vi "AI@InstanceEditor__Parameter.vi"(1 "ParamterIn":string) -> (0 "ParamterOut":string)   [LabVIEW 2020]
uses:
  MainFrame/Global.vi
  <vilib>/vision/NI_Vision_Development_Module.lvlib
panel:
  in  "Rotate":string(combo)
  out "Image":T1(plugin-control)
  in  "Preview":bool
  in  "SubDir":string(combo)
  in  "Capture":string(combo)
  in  "Confirm":bool
  # "AI@InstanceEditor $Capture(\\$Directory)(,Rotate=1)"
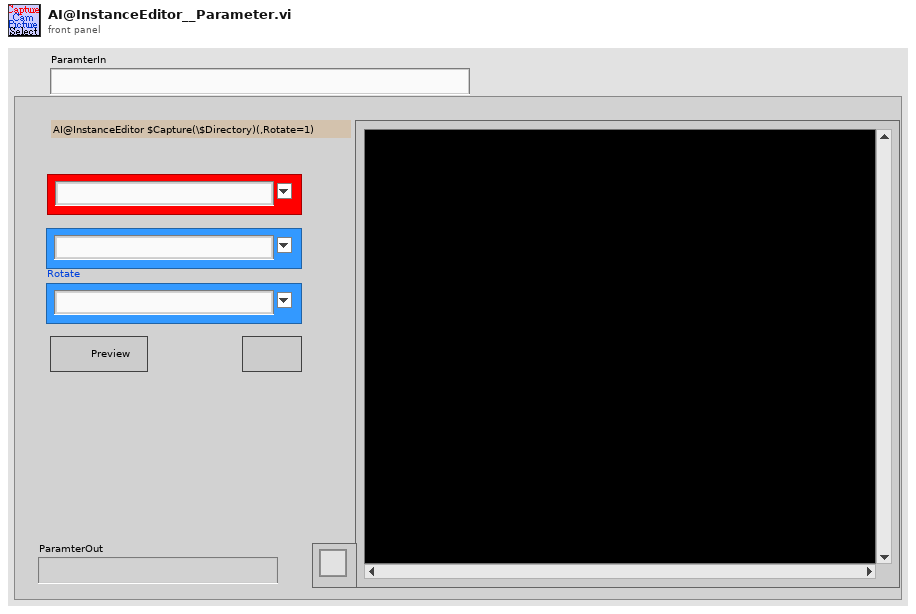
[diagram p1: front panel]
types:
  T1 = typedef "IMAQ Image.ctl" = refnum<image>
  T2 = cluster{"Browser Size":cluster{"X":i32, "Y":i32}, "Images per Line":i32, "Background Color":u32, "Frame Size":i32, "Frame Style":u16}
  T3 = typedef "Image Type" = u32
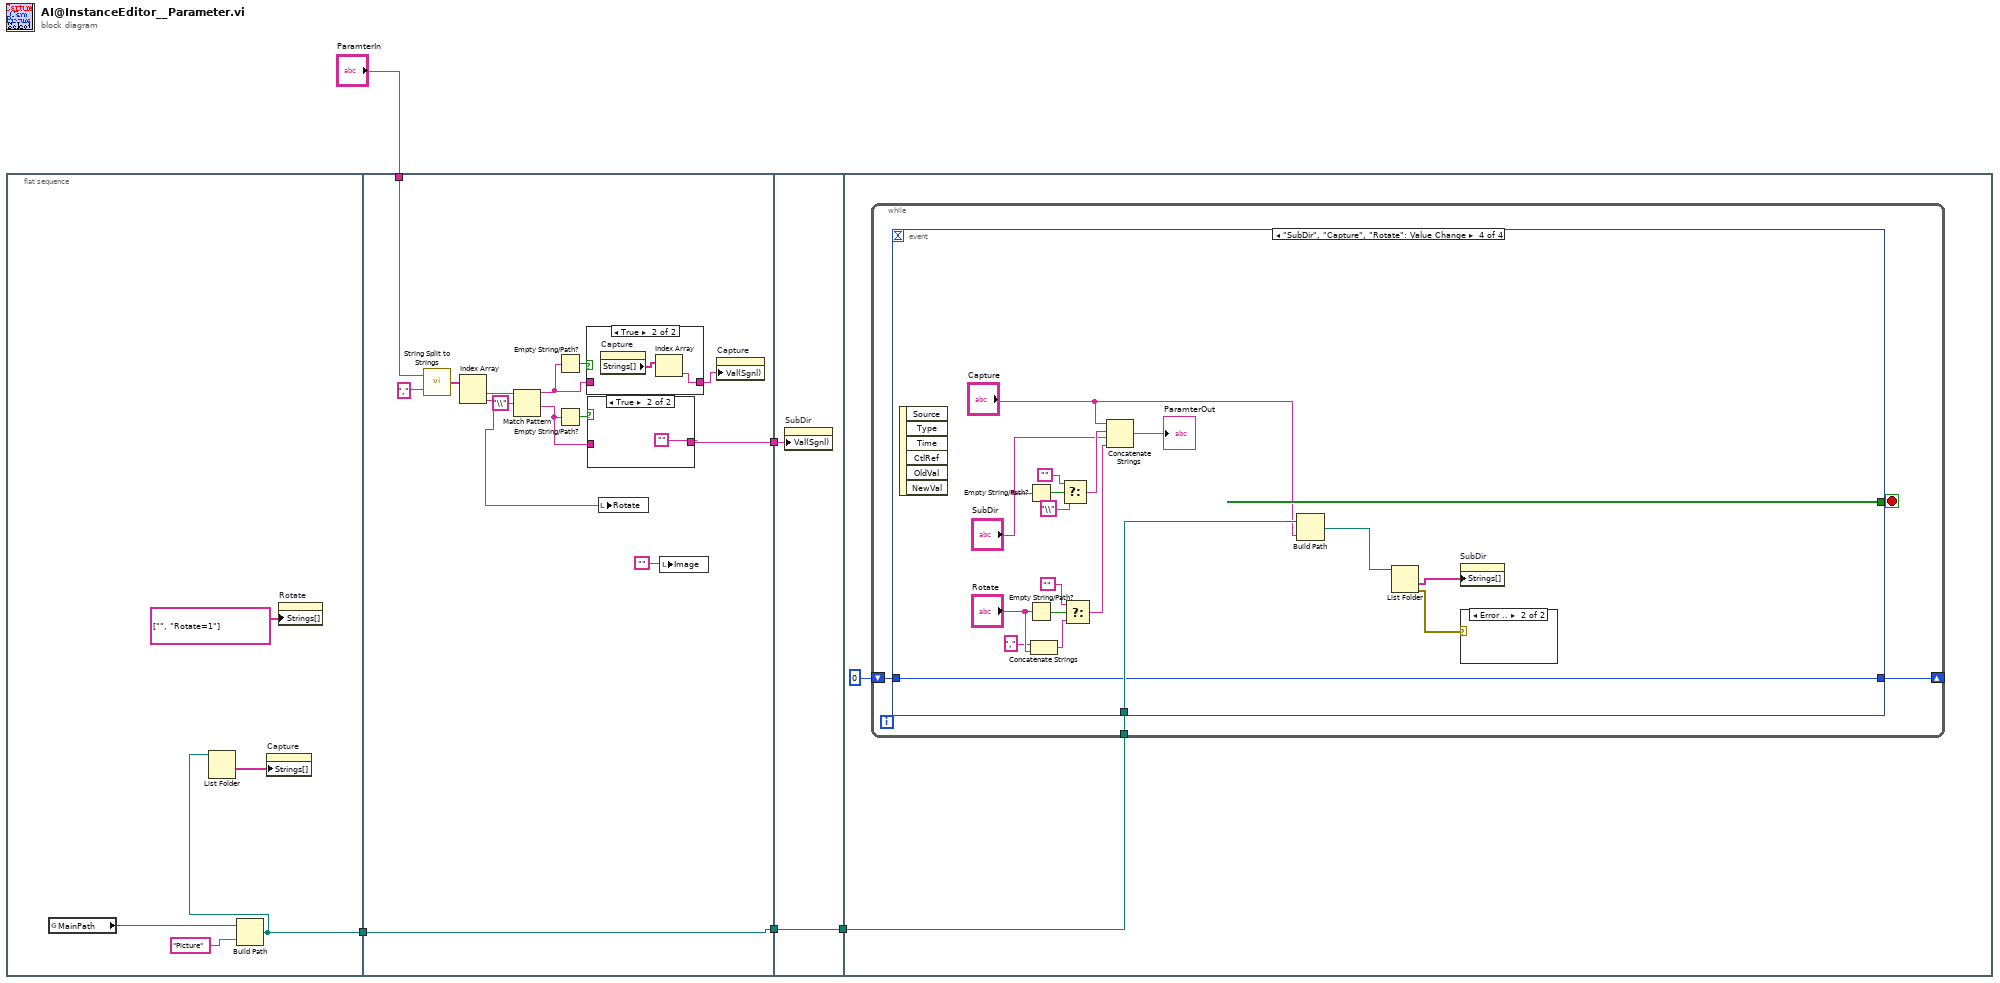
[diagram p0: block diagram]
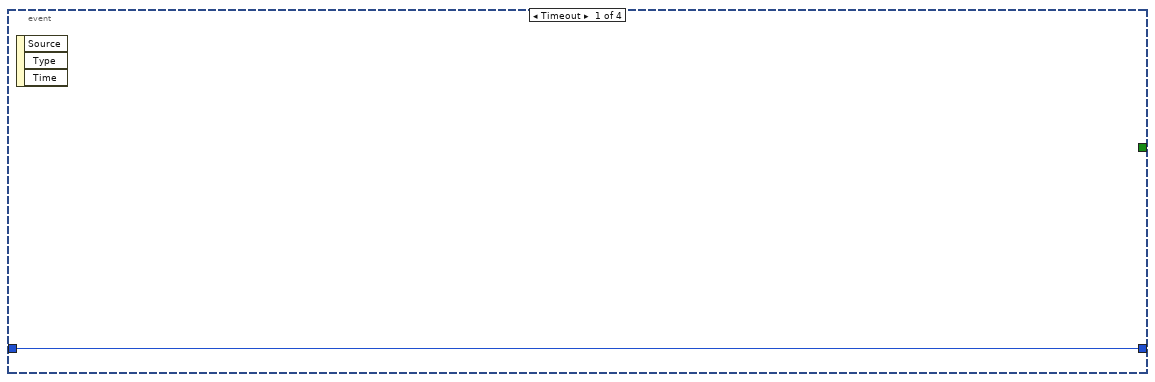
[diagram p4: hidden frame]
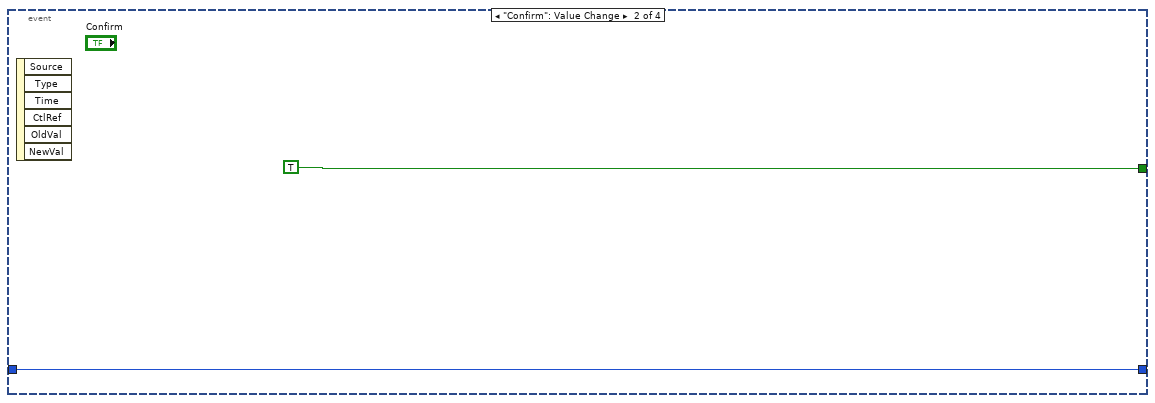
[diagram p5: hidden frame]
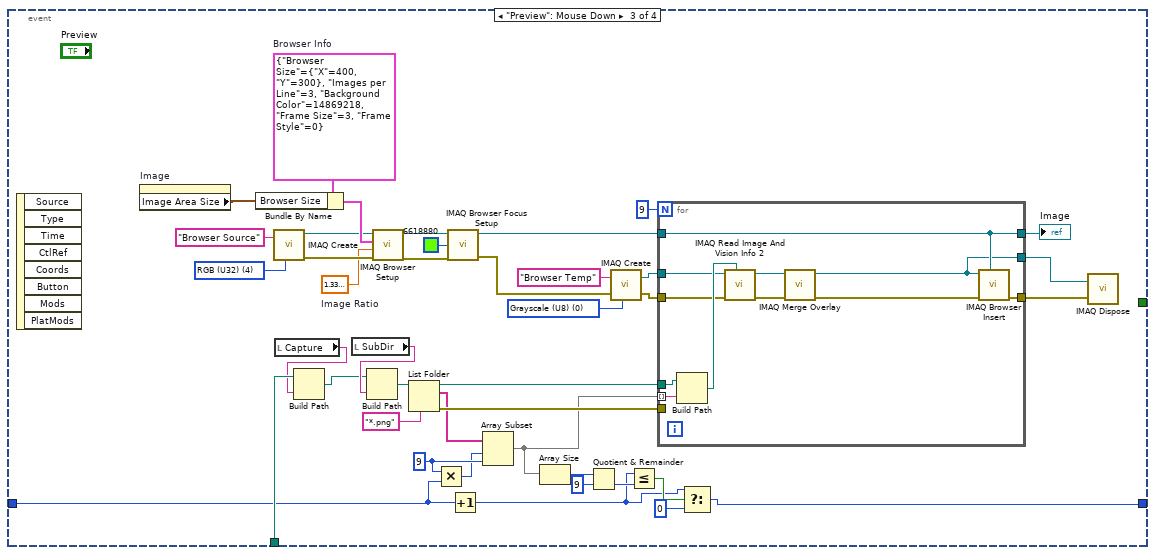
[diagram p6: hidden frame]
diagram:
  n1 = flat-sequence {
    tunnel: [w8] -> w2
    tunnel: "ParamterIn" -> [w22]
    tunnel: [w20] -> w3
    tunnel: w2 -> [w20]
    tunnel: [w19] -> w1
    tunnel: [w31] -> w4
    tunnel: w3 -> [w31]
    tunnel: w1 -> [w30]
    tunnel: w4 -> [w33]
    frame #0 {
      n2 = global read "Global.vi" "MainPath"() -> (w9:path)
      n3 = Build Path(base path=w9, name or relative path="Picture") -> (appended path=w8:path)
      n4 = List Folder(path=w8) -> (folder names=w7:string[])  [unwired: 3 in, 3 out]
      n5 = property on="Capture" class="CmbBox"("Strings[]"=w7) -> ()  [unwired: 2 in, 2 out]
      n6 = property on="Rotate" class="CmbBox"("Strings[]"=string[] ["", "Rotate=1"] ("Strings []")) -> ()  [unwired: 2 in, 2 out]
    }
    frame #1 {
      n7 = call "String Split to Strings.vi"("search string/char (-)"=",", "String"=w22) -> ("Array"=w24:string[])
      n8 = Index Array(array=w24) -> (element #1=w16:string, element #2=w11:string)  [unwired: 2 in]
      n9 = Match Pattern(string=w16, regular expression="\\") -> (before substring=w14:string, after substring=w13:string)  [unwired: 1 in, 2 out]
      n10 = Empty String/Path?(string/path=w14) -> (empty?=w21:bool)
      n11 = Empty String/Path?(string/path=w13) -> (empty?=w17:bool)
      n12 = case shown="True" w21 {
        tunnel: w14 -> [w27 _]
        tunnel: [w27 w28] -> w18
        frame False {
        }
        frame True {
          n13 = property on="Capture" class="CmbBox"() -> ("Strings[]"=w29:string[])  [unwired: 2 in, 2 out]
          n14 = Index Array(array=w29) -> (element=w28:string)  [unwired: 1 in]
        }
      }
      n15 = case shown="True" w17 {
        tunnel: [w25 ""] -> w19
        tunnel: w13 -> [w25 _]
        frame False {
        }
        frame True {
        }
      }
      n16 = local write "Rotate"(w11) -> ()
      n17 = local write "Image"("") -> ()
      n18 = property on="Capture" class="CmbBox"("Val(Sgnl)"=w18) -> ()  [unwired: 2 in, 2 out]
    }
    frame #2 {
      n19 = property on="SubDir" class="CmbBox"("Val(Sgnl)"=w30) -> ()  [unwired: 2 in, 2 out]
    }
    frame #3 {
      n20 = while {
        tunnel: w33 -> [w36]
        shift-right: [w34] -> _
        shift-left: 0 -> [w35]
        stop <- w37 stop-if-true
        n21 = event shown="[3] \"SubDir\", \"Capture\", \"Rotate\": Value Change" {
          selector: _ -> [_ _ _ _]
          dyn-events: _ -> [_ _ _ _]
          timeout: _ -> [_ _ _ _]
          tunnel: [_ TRUE _ _] -> w37
          tunnel: w36 -> [_ _ w56 w108]
          tunnel: w35 -> [w38 w39 w50 w99]
          tunnel: [w38 w39 w42 w99] -> w34
          event Timeout {
            n22 = event-data() -> ()  [unwired: 1 in, 3 out]
          }
          event "Confirm": Value Change {
            n23 = event-data() -> ()  [unwired: 1 in, 6 out]
          }
          event "Preview": Mouse Down {
            w52 = 9 ("length")
            w60 = sgl 1.33  # Image Ratio
            w77 = T2 {"Browser Size"={"X"=400, "Y"=300}, "Images per Line"=3, "Background Color"=14869218, "Frame Size"=3, "Frame Style"=0}  # Browser Info
            w68 = T3 0 items=["Grayscale (U8)", "Grayscale (I16)", "Grayscale (SGL)", "Complex (CSG)", "RGB (U32)", "HSL (U32)", "RGB (U64)", "Grayscale (U16)"] ("Image Type")
            w66 = T3 4 items=["Grayscale (U8)", "Grayscale (I16)", "Grayscale (SGL)", "Complex (CSG)", "RGB (U32)", "HSL (U32)", "RGB (U64)", "Grayscale (U16)"] ("Image Type")
            n24 = event-data() -> ()  [unwired: 1 in, 8 out]
            n25 = property on="Image" class="ImageControl"() -> ("Image Area Size"=w78:cluster{"Width":u32, "Height":u32})  [unwired: 2 in, 2 out]
            n26 = Bundle By Name(cluster=w77, "Browser Size"=w78) -> (w79:T2)
            n27 = call "IMAQ Create"("Image Name"="Browser Source", "Image Type"=w66) -> ("New Image"=w64:T1, "error out"=w65:errorcluster)  [unwired: 3 in]
            n28 = local read "Capture"() -> (w55:string)
            n29 = Build Path(base path=w56, name or relative path=w55) -> (appended path=w54:path)
            n30 = local read "SubDir"() -> (w59:string)
            n31 = Build Path(base path=w54, name or relative path=w59) -> (appended path=w58:path)
            n32 = call "IMAQ Browser Setup"("error in (no error)"=w65, "Image Ratio"=w60, "Browser Info"=w79, "Image In"=w64) -> ("error out"=w73:errorcluster, "Image Browser Out"=w72:T1)  [unwired: 2 out]
            n33 = List Folder(path=w58, pattern="*.png") -> (path out=w63:path, filenames=w41:string[], error out=w80:errorcluster)  [unwired: 2 in, 1 out]
            n34 = Multiply(x=w52, y=w50) -> (x*y=w51:i32)
            n35 = call "IMAQ Browser Focus Setup"("error in (no error)"=w73, "Focus Color"=u32 6618880, "Image Browser In"=w72) -> ("error out"=w75:errorcluster, "Image Browser Out"=w74:T1)  [unwired: 1 in]
            n36 = Increment(x=w50) -> (x+1=w44:i32)
            n37 = Array Subset(array=w41, index=w51, length=w52) -> (w49:string[])
            n38 = Array Size(array=w49) -> (size(s)=w48:i32)
            n39 = Quotient & Remainder(x=w48, y=9) -> (floor(x/y)=w46:i32)  [unwired: 1 out]
            n40 = call "IMAQ Create"("Image Name"="Browser Temp", "Image Type"=w68, "error in (no error)"=w75) -> ("New Image"=w70:T1, "error out"=w61:errorcluster)  [unwired: 2 in]
            n41 = Less Or Equal?(x=w44, y=w46) -> (x <= y?=w45:bool)
            n42 = for {
              N: 9 -> [_]
              tunnel: w74 -> [w87]
              tunnel: w63 -> [w92]
              tunnel: w61 -> [w90]
              tunnel: [w89] -> w62
              tunnel: [w87] -> w81
              tunnel: w70 -> [w88]
              tunnel: [w84] -> w71
              tunnel: w80 -> [_]
              tunnel: w49 -> [w82] mode=indexing
              n43 = Build Path(base path=w92, name or relative path=w82) -> (appended path=w91:path)
              n44 = call "IMAQ Read Image And Vision Info 2"("File Path"=w91, "error in (no error)"=w90, "Image"=w88) -> ("error out"=w86:errorcluster, "Image Out"=w85:T1)  [unwired: 6 in, 1 out]
              n45 = call "IMAQ Merge Overlay"("error in (no error)"=w86, "Image Src"=w85) -> ("error out"=w83:errorcluster, "Image Dst Out"=w84:T1)  [unwired: 8 in]
              n46 = call "IMAQ Browser Insert"("Image Browser In"=w87, "error in (no error)"=w83, "Image to Add"=w84) -> ("error out"=w89:errorcluster)  [unwired: 4 in, 4 out]
            }
            "Image" <- w81
            n47 = Select(t=w44, s=w45, f=0) -> (s? t:f=w42:i32)
            n48 = call "IMAQ Dispose"("Image"=w71, "error in (no error)"=w62) -> ()  [unwired: 4 in, 1 out]
          }
          event "SubDir", "Capture", "Rotate": Value Change {
            n49 = event-data() -> ()  [unwired: 1 in, 6 out]
            n50 = Empty String/Path?(string/path="SubDir") -> (empty?=w104:bool)
            n51 = Empty String/Path?(string/path="Rotate") -> (empty?=w98:bool)
            n52 = Concatenate Strings("," ("string"), "Rotate") -> (w94:string)
            n53 = Select(t="", s=w104, f="\\" ("string")) -> (s? t:f=w101:string)
            n54 = Select(t="", s=w98, f=w94) -> (s? t:f=w93:string)
            n55 = Concatenate Strings("Capture", w101, "SubDir", w93) -> (→"ParamterOut":string)
            n56 = Build Path(base path=w108, name or relative path="Capture") -> (appended path=w107:path)
            n57 = List Folder(path=w107) -> (folder names=w106:string[], error out=w109:errorcluster)  [unwired: 3 in, 2 out]
            n58 = property on="SubDir" class="CmbBox"("Strings[]"=w106) -> ()  [unwired: 2 in, 2 out]
            n59 = case shown="Error .." w109 {
              frame No Error {
              }
              frame Error {
              }
            }
          }
        }
      }
    }
  }
